vi "Init.vi"(8 "error in":errorcluster, 11 "Alarming Strategy in":refnum<class "Alarming Actor Strategy.lvclass">) -> (0 "error out":errorcluster, 3 "Alarming Strategy out":refnum<class "Alarming Actor Strategy.lvclass">)   [LabVIEW 2024, in "Alarming Actor Strategy.lvclass"]
uses:
  Alarming Actor Strategy.lvclass
  Alarming Actor Strategy.lvclass/Alarming Actor Strategy.ctl
  <vilib>/ActorFramework/Actor/Actor.lvclass
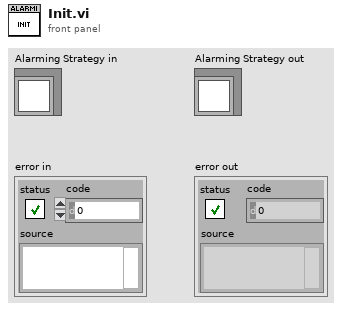
[diagram p1: front panel]
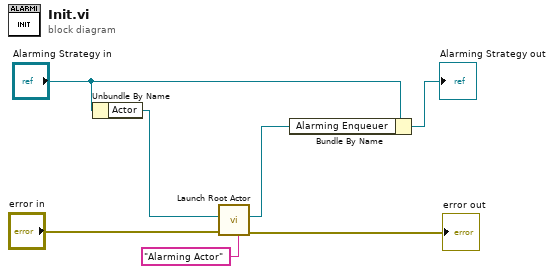
[diagram p0: block diagram]
diagram:
  n1 = Unbundle By Name("Alarming Strategy in") -> ("Actor"=w1:refnum<class "Actor.lvclass">)
  n2 = call <vilib>:"Launch Root Actor.vi"("Debug Alias"="Alarming Actor", "error in (no error)"="error in", "Actor"=w1) -> ("error out"=→"error out":errorcluster, "Actor's Enqueuer"=w7:refnum<class "Message Enqueuer.lvclass">)  [unwired: 7 in]
  n3 = Bundle By Name(cluster="Alarming Strategy in", "Alarming Enqueuer"=w7) -> (→"Alarming Strategy out":refnum<class "Alarming Actor Strategy.lvclass">)
